vi "DestroyPriorityQueue.vi"(8 "error in (no error)":errorcluster, 11 "Queue":refnum<data-value>) -> (0 "error out":errorcluster)   [LabVIEW 2009, in "PriorityQueue.lvclass"]
uses:
  PriorityQueue.lvclass
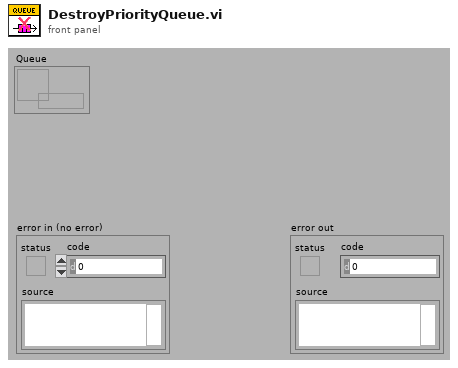
[diagram p1: front panel]
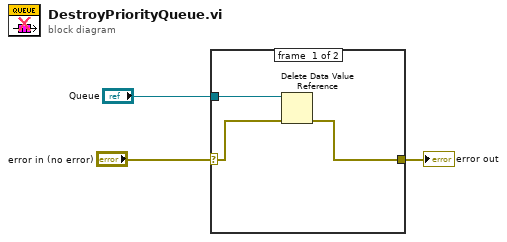
[diagram p0: block diagram]
diagram:
  n1 = case shown="No Error" "error in (no error)" {
    selector: "error in (no error)" -> [w4 w7]
    tunnel: "Queue" -> [w6 _]
    tunnel: [w5 w7] -> w2
    frame #0 {
      n2 = Delete Data Value Reference(data value reference=w6, error in=w4) -> (error out=w5:errorcluster)  [unwired: 1 out]
    }
    frame #1 {
    }
  }
  "error out" <- w2
